vi "Arrays.vi"() -> ()   [LabVIEW 2014]
panel:
  in  "stop":bool
  out "Array 4":bool[](array[boolean])
  out "Array 3":dbl[](array[slide]) scale=0.0..10.0
  in  "Array 2":bool[](array[boolean])
  in  "Array":dbl[](array[numeric])
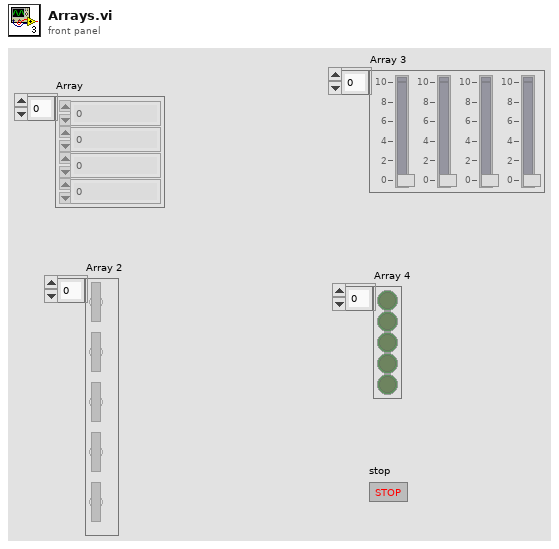
[diagram p1: front panel]
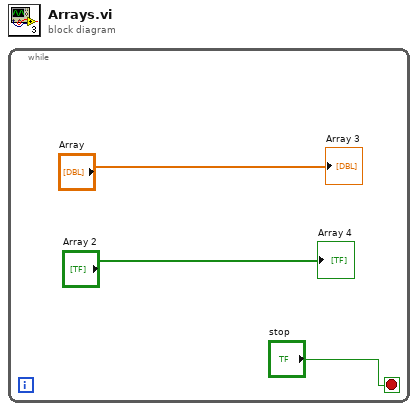
[diagram p0: block diagram]
diagram:
  n1 = while {
    stop <- "stop" stop-if-true
    "Array 3" <- "Array"
    "Array 4" <- "Array 2"
  }
